vi "Create DO Task.vi"(8 "error in (no error)":errorcluster, 11 "DO Channel Setting":T1) -> (0 "error out":errorcluster, 3 "DO_Task":refnum<k21>)   [LabVIEW 2016, in "DAQ IO.lvlib"]
uses:
  DAQ IO.lvlib
  DO Channel Setting.ctl
  <vilib>/DAQmx/create/channels.llb/DAQmx Create Channel (DO-Digital Output).vi
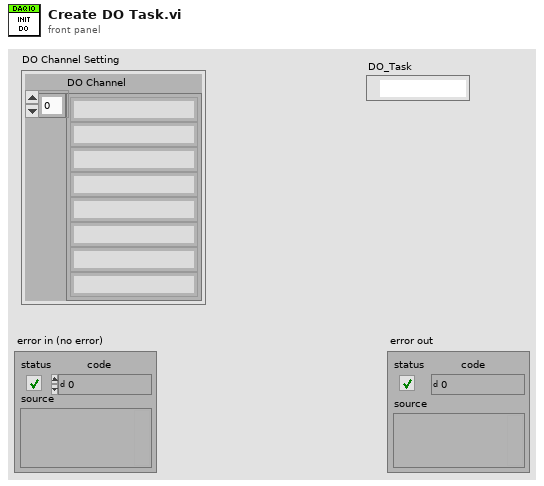
[diagram p1: front panel]
types:
  T1 = typedef "DAQ IO.lvlib/DO Channel Setting.ctl" = cluster{"DO Channel":string[]}
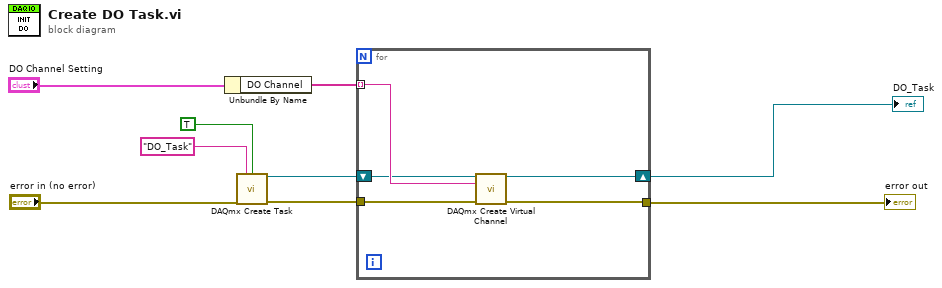
[diagram p0: block diagram]
diagram:
  n1 = Unbundle By Name("DO Channel Setting") -> ("DO Channel"=w7:string[])
  n2 = call <vilib>:"DAQmx Create Task.vi"("new task name"="DO_Task" ("name to assign"), "auto cleanup"=TRUE, "error in"="error in (no error)") -> ("task out"=w5:refnum<k21>, "error out"=w8:errorcluster)  [unwired: 11 in]
  n3 = for {
    tunnel: w8 -> [w14]
    tunnel: w7 -> [w11] mode=indexing
    tunnel: [w13] -> w3
    shift-right: [w12] -> w2
    shift-left: w5 -> [w10]
    n4 = call-poly <vilib>:"DAQmx Create Virtual Channel.vi"("task in"=w10, "Lines"=w11, "error in"=w14) -> ("task out"=w12:refnum<k21>, "error out"=w13:errorcluster)  [unwired: 11 in]
  }
  "error out" <- w3
  "DO_Task" <- w2
